vi "Configure IQ Recorder Measurement Magnitude Unit.vi"(8 "error in (no error)":errorcluster, 9 "Magnitude Unit (Voltage unit)":i32(ring) items=["Voltage unit", "Raw I/Q data"], 10 "Instance (1)":i32=1, 11 "VISA resource name":refnum<visa-resource-name>) -> (0 "error out":errorcluster, 3 "VISA resource name out":refnum<visa-resource-name>)   [LabVIEW 2015, in "Rohde&Schwarz CMXP GPRF.lvlib"]
doc: "Selets the magnitude unit for the measurement results.\n\nAttribute:\nRSCMXPGPRF_ATTR_IQ_RECORDER_MEASUREMENT_MAGNITUDE_UNIT\n\nRemote-control command:\nCONFigure:GPRF:MEAS<i>:IQRecorder:MUNit"
uses:
  <instrlib>/Rohde&Schwarz CMXP GPRF/Rohde&Schwarz CMXP GPRF.lvlib
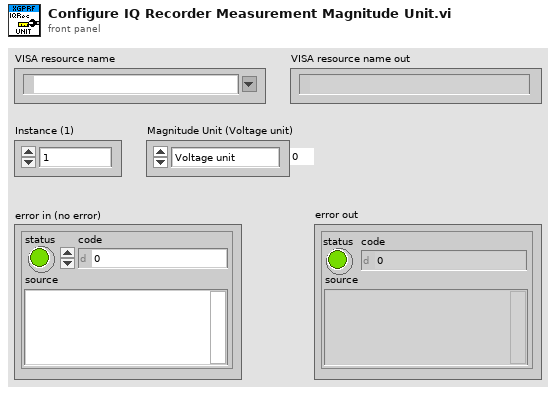
[diagram p1: front panel]
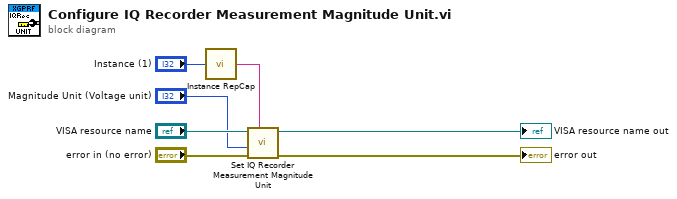
[diagram p0: block diagram]
diagram:
  n1 = call <instrlib>:"Instance RepCap.vi"("instance  in"="Instance (1)") -> ("instance out"=w4:string)
  n2 = call "Set IQ Recorder Measurement Magnitude Unit"("Repeated Capabilities"=w4, "error in (no error)"="error in (no error)", "IQ Recorder Measurement Magnitude Unit (0 - Voltage unit)"="Magnitude Unit (Voltage unit)", "instrument handle"="VISA resource name") -> ("error out"=→"error out":errorcluster, "instrument handle out"=→"VISA resource name out":refnum<visa-resource-name>)  [unwired: 6 in]
